vi "QTMCommander.vi"(4 "Error In":errorcluster) -> ()   [LabVIEW 2017]
uses:
  Globals/QualisysInstruction.vi
  <userlib>/QLC/QLC.lvlib
panel:
  in  "Control QTM":bool=TRUE
  in  "stop":bool
  out "Numeric 2":i32
  out "LoopTime 2":u32(graph)
  out "LoopTime":u32(graph)
  out "Numeric":i32
  in  "Send Trig":bool
  in  "Stop Capture":bool
  in  "Close Measurement":bool
  in  "New Measurement":bool caption="Start Measurement"
  in  "Start Capture":bool
  out "Camera Timestamp":u64
  out "Camera Frame Num":u32
  out "Controlling QTM":bool
  out "Last QTM Event":dbl=2.0
  out "QTM Message":string
  # "Qualisys Commander"
  # "Qualisys commands"
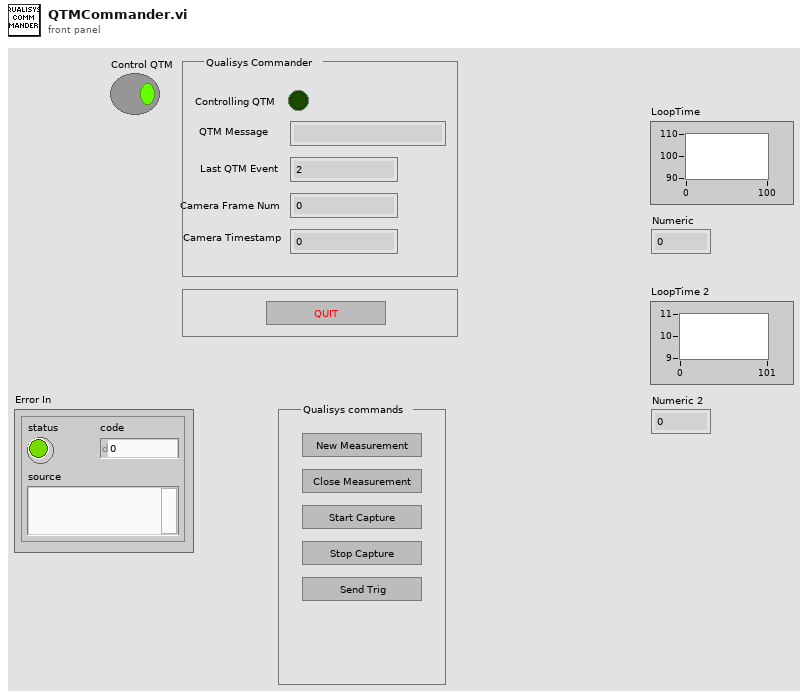
[diagram p1: front panel]
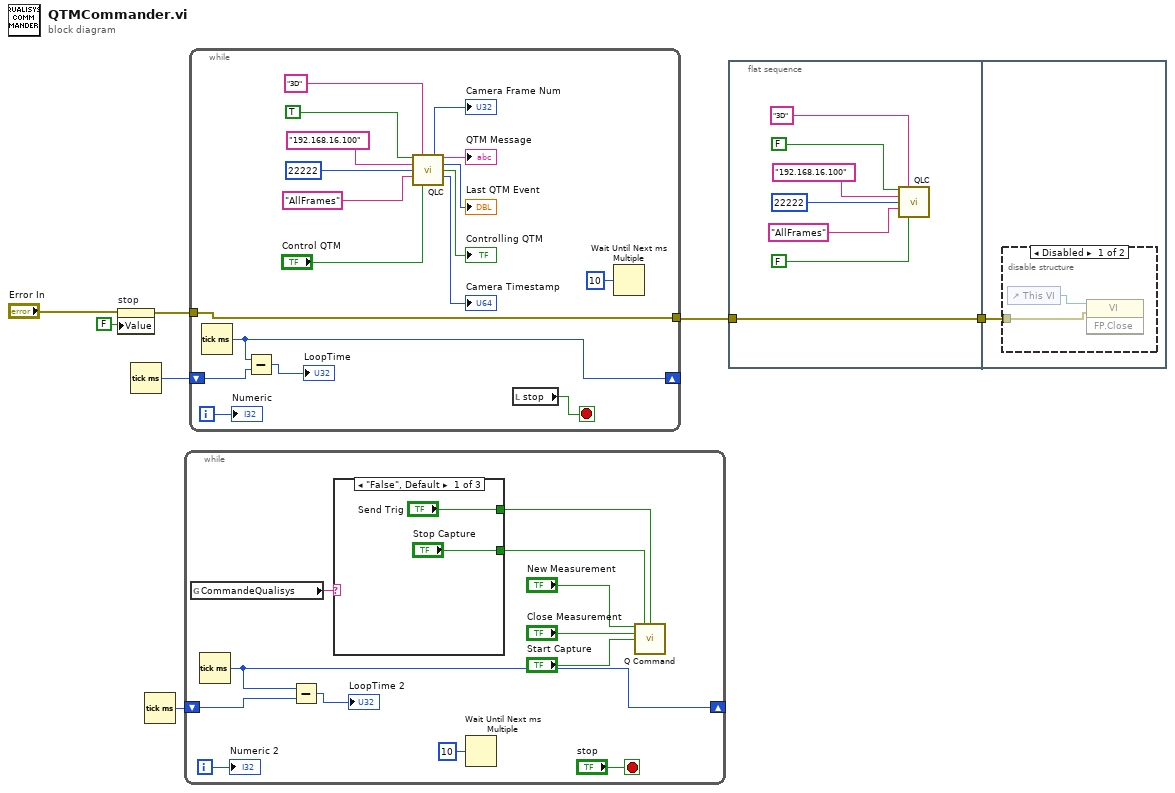
[diagram p0: block diagram]
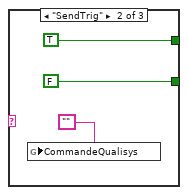
[diagram p2: hidden frame]
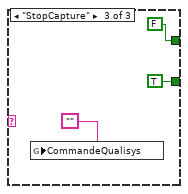
[diagram p3: hidden frame]
diagram:
  n1 = property on="stop" class="Bool (strict)"(error in="Error In", "Value"=FALSE ("stop")) -> (error out=w6:errorcluster)  [unwired: 1 in, 1 out]
  n2 = Tick Count (ms)() -> (millisecond timer value=w7:u32)
  n3 = Tick Count (ms)() -> (millisecond timer value=w1:u32)
  n4 = while {
    shift-right: [w16] -> _
    shift-left: w1 -> [w17]
    i -> [w18]
    stop <- "stop" stop-if-true
    n5 = global read "QualisysInstruction.vi" "CommandeQualisys"() -> (w11:string)
    n6 = Tick Count (ms)() -> (millisecond timer value=w16:u32)
    n7 = Subtract(x=w16, y=w17) -> (x-y=→"LoopTime 2":u32)
    n8 = case shown="\"False\", Default" w11 {
      tunnel: ["Send Trig" TRUE ("Send Trig") FALSE ("Send Trig")] -> w10
      tunnel: ["Stop Capture" FALSE ("Stop Capture") TRUE ("Stop Capture")] -> w9
      frame "False", Default {
      }
      frame "SendTrig" {
        n9 = global write "QualisysInstruction.vi" "CommandeQualisys"("") -> ()
      }
      frame "StopCapture" {
        n10 = global write "QualisysInstruction.vi" "CommandeQualisys"("") -> ()
      }
    }
    n11 = Wait Until Next ms Multiple(millisecond multiple=u32 10) -> ()  [unwired: 1 out]
    n12 = call <userlib>:"Q Command.vi"("bNew"="New Measurement", "bStop"=w9, "bTrig"=w10, "bClose"="Close Measurement", "bStart"="Start Capture") -> ()  [unwired: 10 in, 1 out]
    "Numeric 2" <- w18
  }
  n13 = while {
    shift-right: [w32] -> _
    shift-left: w7 -> [w33]
    tunnel: w6 -> [w28]
    tunnel: [w28] -> w3
    i -> [w34]
    stop <- w29 stop-if-true
    n14 = Tick Count (ms)() -> (millisecond timer value=w32:u32)
    n15 = Subtract(x=w32, y=w33) -> (x-y=→"LoopTime":u32)
    n16 = call <userlib>:"QLC.vi"("connect"=TRUE ("Connect to QTM"), "data"="3D" ("Data"), "address"="192.168.16.100" ("Address"), "port"=22222 ("Port"), "frequency"="AllFrames" ("Frequency"), "controlQTM"="Control QTM") -> ("camFrameNumber"=→"Camera Frame Num":u32, "message"=→"QTM Message":string, "lastEvent"=→"Last QTM Event":i32, "QTMMaster"=→"Controlling QTM":bool, "camTimeStamp"=→"Camera Timestamp":u64)  [unwired: 4 in, 1 out]
    n17 = local read "stop"() -> (w29:bool)
    n18 = Wait Until Next ms Multiple(millisecond multiple=u32 10) -> ()  [unwired: 1 out]
    "Numeric" <- w34
  }
  n19 = flat-sequence {
    tunnel: w3 -> [w52]
    tunnel: [w52] -> w2
    tunnel: w2 -> [w53]
    frame #0 {
      n20 = call <userlib>:"QLC.vi"("connect"=FALSE ("Connect to QTM"), "data"="3D" ("Data"), "address"="192.168.16.100" ("Address"), "port"=22222 ("Port"), "frequency"="AllFrames" ("Frequency"), "controlQTM"=FALSE ("Control QTM")) -> ()  [unwired: 4 in, 6 out]
    }
    frame #1 {
      n21 = disable-structure shown="Disabled" {
        disable-tunnel: w53 -> [w54 _]
        frame Disabled {
          n22 = control-ref of="This VI"() -> (w55:refnum<vi>)
          n23 = invoke class="VI" method="FP.Close"(reference=w55, error in=w54) -> ()  [unwired: 1 in, 3 out]
        }
        frame Enabled {
        }
      }
    }
  }
